vi "RaiseForTime.vi"() -> ()   [LabVIEW 2018]
uses:
  Framework/Robot Global Data.vi
panel:
  in  "NoWait":bool
  in  "Speed":dbl
  in  "Time":dbl
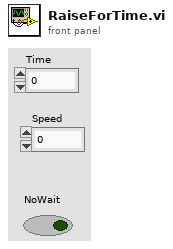
[diagram p1: front panel]
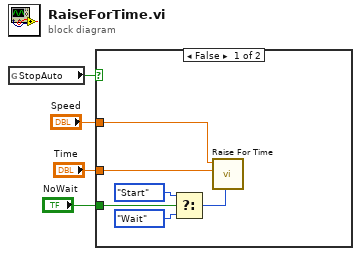
[diagram p0: block diagram]
diagram:
  n1 = global read "Robot Global Data.vi" "StopAuto"() -> (w4:bool)
  n2 = case shown="False" w4 {
    tunnel: "Time" -> [w5 _]
    tunnel: "Speed" -> [w6 _]
    tunnel: "NoWait" -> [w8 _]
    frame False {
      n3 = Select(t=enum16{"Start", "Wait"}."Start" ("Synchronization"), s=w8, f=enum16{"Start", "Wait"}."Wait" ("Synchronization")) -> (s? t:f=w7:enum16{"Start", "Wait"})
      n4 = call "Raise For Time.vi"("Synchronization"=w7, "Time"=w5, "Speed"=w6) -> ()  [unwired: 8 in, 1 out]
    }
    frame True {
    }
  }
